vi "acquire single init subvi.vi"(8 "error in":errorcluster, 11 "VISA resource name":refnum<visa-resource-name>) -> (0 "error out":errorcluster, 1 "index":i32, 2 "read buffer":string, 3 "VISA resource name out":refnum<visa-resource-name>)   [LabVIEW 2023, in "owon.lvlib"]
uses:
  owon.lvlib
panel:
  out "ID query resp":string
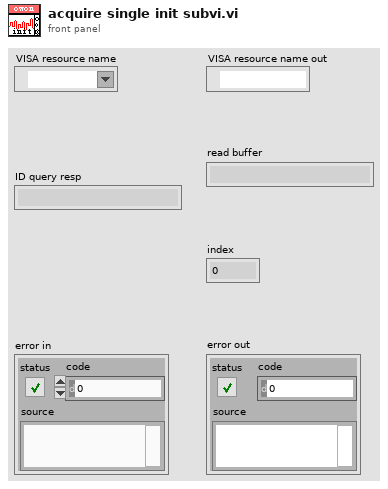
[diagram p1: front panel]
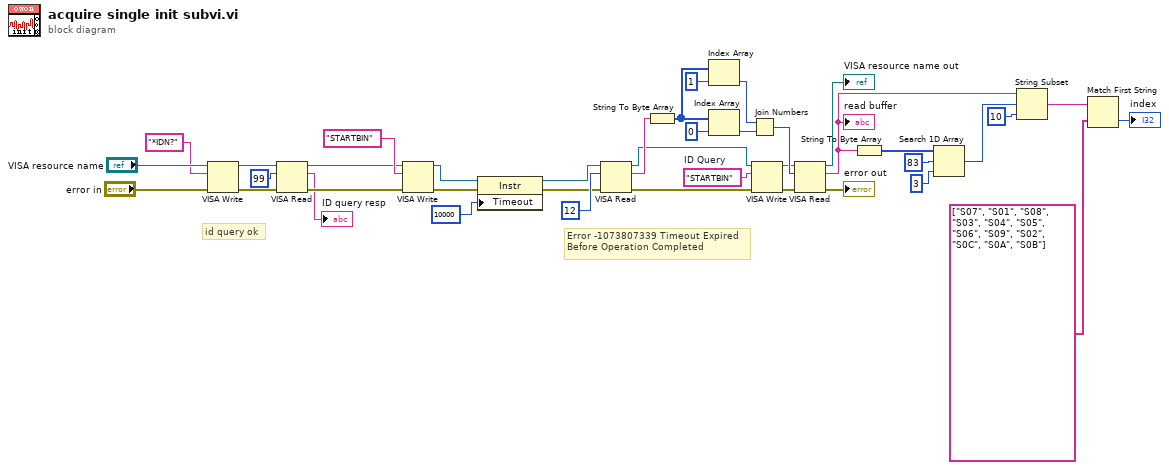
[diagram p0: block diagram]
diagram:
  w28 = "STARTBIN"  # ID Query
  # "Error -1073807339 Timeout Expired\nBefore Operation Completed"
  # "id query ok"
  n1 = VISA Write(VISA resource name="VISA resource name", write buffer="*IDN?", error in (no error)="error in") -> (VISA resource name out=w8:refnum<visa-resource-name>, error out=w12:errorcluster)  [unwired: 1 out]
  n2 = VISA Read(VISA resource name=w8, byte count=u32 99, error in (no error)=w12) -> (VISA resource name out=w7:refnum<visa-resource-name>, read buffer=→"ID query resp":string, error out=w9:errorcluster)  [unwired: 1 out]
  n3 = VISA Write(VISA resource name=w7, write buffer="STARTBIN" ("Start Measurement"), error in (no error)=w9) -> (VISA resource name out=w38:refnum<visa-resource-name>, error out=w3:errorcluster)  [unwired: 1 out]
  n4 = property class="Instr"(reference=w38, error in=w3, "Timeout"=u32 10000 ("General Settings:Timeout Value")) -> (reference out=w4:refnum<visa-resource-name>, error out=w2:errorcluster)
  n5 = VISA Read(VISA resource name=w4, byte count=u32 12, error in (no error)=w2) -> (VISA resource name out=w29:refnum<visa-resource-name>, read buffer=w32:string, error out=w30:errorcluster)  [unwired: 1 out]
  n6 = String To Byte Array(string=w32) -> (unsigned byte array=w33:u8[])
  n7 = Index Array(array=w33, index=1 ("索引")) -> (element=w36:u8)
  n8 = Index Array(array=w33, index=0 ("索引")) -> (element=w37:u8)
  n9 = Join Numbers(hi=w36, lo=w37) -> ((hi.lo)=w39:u16)
  n10 = VISA Write(VISA resource name=w29, write buffer=w28, error in (no error)=w30) -> (VISA resource name out=w26:refnum<visa-resource-name>, error out=w27:errorcluster)  [unwired: 1 out]
  n11 = VISA Read(VISA resource name=w26, byte count=w39, error in (no error)=w27) -> (VISA resource name out=→"VISA resource name out":refnum<visa-resource-name>, read buffer=w19:string, error out=→"error out":errorcluster)  [unwired: 1 out]
  "read buffer" <- w19
  n12 = String To Byte Array(string=w19) -> (unsigned byte array=w18:u8[])
  n13 = Search 1D Array(1D array=w18, element=u8 83 ("元素"), start index (0)=3 ("开始索引(0)")) -> (index of element=w15:i32)
  n14 = String Subset(string=w19, offset (0)=w15, length (rest)=10 ("长度（剩余）")) -> (substring=w22:string)
  n15 = Match First String(2:string[] ["S07", "S01", "S08", "S03", "S04", "S05", "S06", "S09", "S02", "S0C", "S0A", "S0B"], 3:w22) -> (0:→"index":i32)  [unwired: 1 out]
